vi "HTDateTimeToSQLDatetime.vi"(10 "HTDateTime":string=" 2015_09_22_08_49_03") -> (0 "time stamp":timestamp, 1 "date string":string, 2 "SQLDateTime":string, 4 "Shift":string)   [LabVIEW 2012]
uses:
  <vilib>/Utility/miscctls.llb/LVDateTimeRec.ctl
panel:
  in  "date time rec":T1
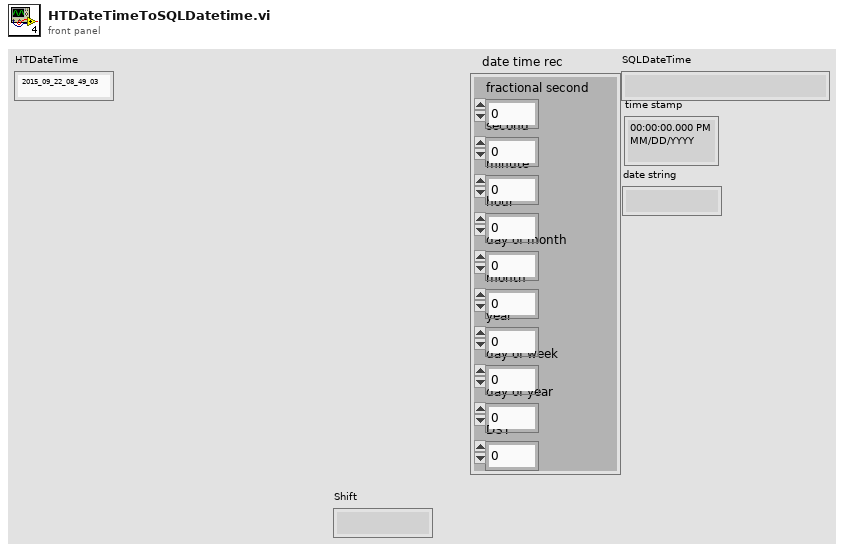
[diagram p1: front panel]
types:
  T1 = typedef "LVDateTimeRec.ctl" = cluster{"fractional second":dbl, "second":i32, "minute":i32, "hour":i32, "day of month":i32, "month":i32, "year":i32, "day of week":i32, "day of year":i32, "DST":i32}
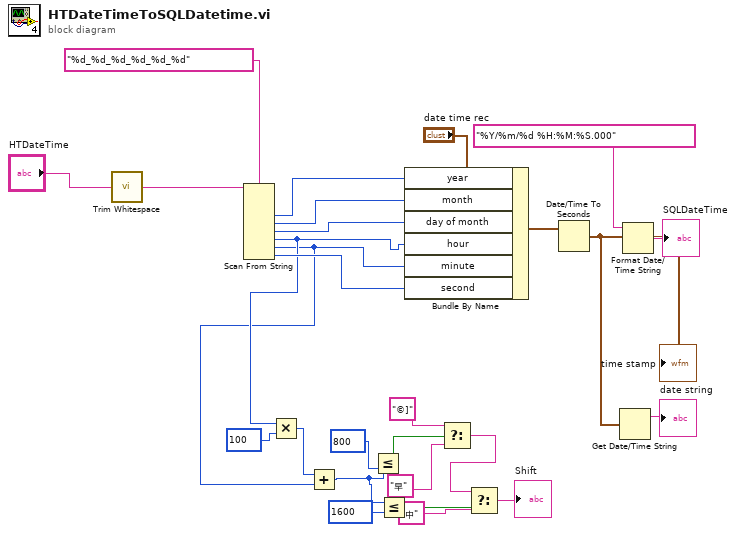
[diagram p0: block diagram]
diagram:
  n1 = call <vilib>:"Trim Whitespace.vi"("string"="HTDateTime") -> ("trimmed string"=w1:string)  [unwired: 1 in]
  n2 = Scan From String(format string="%d_%d_%d_%d_%d_%d", input string=w1) -> (output 1=w25:i32, output 2=w24:i32, output 3=w23:i32, output 4=w4:i32, output 5=w3:i32, output 6=w22:i32)  [unwired: 8 in, 3 out]
  n3 = Multiply(x=w4, y=100) -> (x*y=w15:i32)
  n4 = Add(x=w15, y=w3) -> (x+y=w8:i32)
  n5 = Less Or Equal?(x=w8, y=800) -> (x <= y?=w5:bool)
  n6 = Less Or Equal?(x=w8, y=1600) -> (x <= y?=w10:bool)
  n7 = Bundle By Name(cluster="date time rec", "year"=w25, "month"=w24, "day of month"=w23, "hour"=w4, "minute"=w3, "second"=w22) -> (w21:T1)
  n8 = Select(t="©]", s=w5, f="早") -> (s? t:f=w7:string)
  n9 = Select(t=w7, s=w10, f="中") -> (s? t:f=→"Shift":string)
  n10 = Date/Time To Seconds(2:w21) -> (0:w18:timestamp)  [unwired: 1 in]
  "time stamp" <- w18
  n11 = Get Date/Time String(seconds (now)=w18) -> (date string=→"date string":string)  [unwired: 2 in, 1 out]
  n12 = Format Date/Time String(time format string (%c)="%Y/%m/%d %H:%M:%S.000", seconds (now)=w18) -> (date/time string=→"SQLDateTime":string)  [unwired: 1 in]
